vi "Stop.vi"(8 "error in (no error)":errorcluster, 11 "VISA resource name":refnum<visa-resource-name>) -> (0 "error out":errorcluster, 3 "VISA resource name out":refnum<visa-resource-name>)   [LabVIEW 2020, in "Control de MaP.lvlib"]
doc: "Stop the motors"
uses:
  Control de MaP.lvlib
  <vilib>/Instr/_visa.llb/VISA Flush IO Buffer Mask.ctl
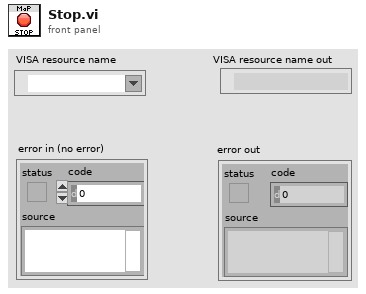
[diagram p1: front panel]
types:
  T1 = typedef "VISA Flush IO Buffer Mask.ctl" = u16
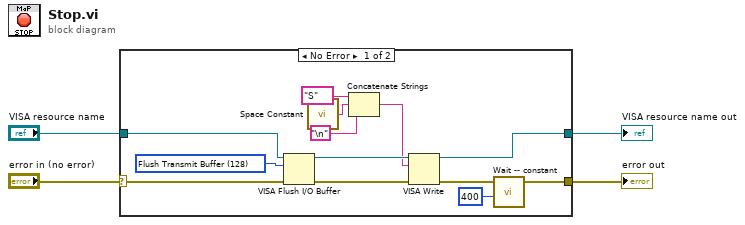
[diagram p0: block diagram]
diagram:
  n1 = case shown="No Error" "error in (no error)" {
    selector: "error in (no error)" -> [w15 w19]
    tunnel: "VISA resource name" -> [w14 w18]
    tunnel: [w17 w18] -> w2
    tunnel: [w10 w19] -> w1
    frame No Error {
      w16 = T1 128 items=["Flush Receive Buffer"=16, "Write Transmit Buffer to Device"=32, "Flush Receive Buffer (No I/O)"=64, "Flush Transmit Buffer"=128] ("Mask")
      n2 = VISA Flush I/O Buffer(VISA resource name=w14, mask (16)=w16, error in (no error)=w15) -> (VISA resource name out=w13:refnum<visa-resource-name>, error out=w12:errorcluster)
      n3 = call <vilib>:"Space Constant.vi"() -> ("String"=w6:string)
      n4 = Concatenate Strings("S" ("write buffer"), w6, "\n") -> (w7:string)
      n5 = VISA Write(VISA resource name=w13, write buffer=w7, error in (no error)=w12) -> (VISA resource name out=w17:refnum<visa-resource-name>, error out=w11:errorcluster)  [unwired: 1 out]
      n6 = call "Wait -- constant.vi"("error in (no error)"=w11, "wait (100 ms)"=u32 400) -> ("error out"=w10:errorcluster)  [unwired: 5 in]
    }
    frame Error {
    }
  }
  "VISA resource name out" <- w2
  "error out" <- w1
